vi "Teleop.vi"(10 "Match Info":T1={"Autonomous Elapsed Seconds"=0.0, "TeleOp Elapsed Seconds"=0.0, "Disabled Elapsed Seconds"=0.0, "Visited Autonomous"=FALSE, "Visited TeleOp"=FALSE, "Visited Disabled"=FALSE, "Autonomous Settings"={"Autonomous Style"=enum."Independent", "VI Refnum"=refnum}}, 11 "Call Context":T2) -> ()   [LabVIEW 2017]
doc: "This VI is called for each TeleOp packet received from the DS where the robot is not disabled. It is often used to read from the joysticks and update I/O or to update setpoints for timed control loops. It should complete and return within 20 milliseconds or it may miss DS packets."
uses:
  <vilib>/Rock Robotics/WPI/DriverStation/WPI_DriverStationDerivedRobotMode.ctl
  <vilib>/Rock Robotics/WPI/DriverStation/WPI_DriverStationMatch Info.ctl
  <vilib>/Rock Robotics/WPI/Utilities/WPI_GetSetVariantRefNum.vi
  <vilib>/Rock Robotics/Network Tables/NT Write Boolean Array.vi
  <vilib>/Rock Robotics/Network Tables/NT Write Numeric Array.vi
  <vilib>/Rock Robotics/Network Tables/NT Read Boolean.vi
  <vilib>/Rock Robotics/Network Tables/NT Read Number.vi
  Robot Global Data.vi
panel:
  out "Sample Slider 0":dbl(slide) scale=0.0..5.0
  out "Sample Boolean 1":bool
  out "Sample Boolean 0":bool
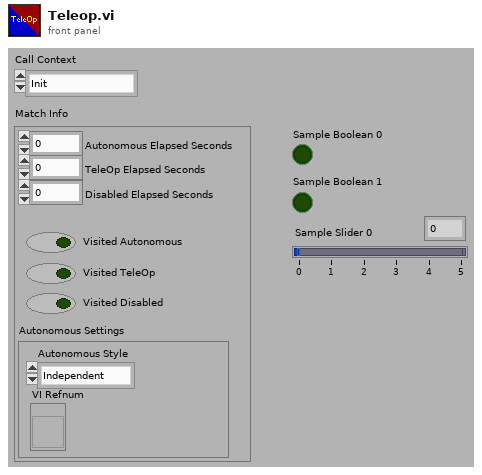
[diagram p1: front panel]
types:
  T1 = typedef "WPI_DriverStationMatch Info.ctl" = cluster{"Autonomous Elapsed Seconds":dbl, "TeleOp Elapsed Seconds":dbl, "Disabled Elapsed Seconds":dbl, "Visited Autonomous":bool, "Visited TeleOp":bool, "Visited Disabled":bool, "Autonomous Settings":cluster{"Autonomous Style":enum16{"Iterative", "Independent"}, "VI Refnum":refnum<vi>}}
  T2 = typedef "WPI_DriverStationDerivedRobotMode.ctl" = enum16{"Init", "Execute", "Stop"}
  T3 = enum16{"Linear", "Square  Root", "Square", "n^x"}
  T4 = typedef "WPI_JoystickDevRef.ctl" = cluster{"Device":T5}
  T5 = typedef "WPI_JoystickDeviceEnum.ctl" = enum16{"USB 0", "USB 1", "USB 2", "USB 3", "USB 4", "USB 5"}
  T6 = typedef "WPI_MotorControlDeviceRef.ctl" = cluster{"DeviceStatus":errorcluster, "Type":T7, "PWM":cluster{"PWM Channel":T8, "DeadBand":T9}, "CAN":cluster{"Device Number":u8, "SetOutput VI Ref":variant, "GetOutput VI Ref":variant, "Enable VI Ref":variant, "Disable VI Ref":variant, "Data":variant}, "Invert":bool, "DIO PWM":cluster{"PWM \"Enable\" Channel":T8, "DIOChannel":T10, "PWM Rate":dbl}}
  T7 = typedef "WPI_MotorControlType.ctl" = enum16{"PWM", "CAN", "DIO PWM"}
  T8 = typedef "FPGA_DIOPWMChannel.ctl" = enum8{"PWM 0", "PWM 1", "PWM 2", "PWM 3", "PWM 4", "PWM 5", "PWM 6", "PWM 7", "PWM 8", "PWM 9", "PWM MXP 0", "PWM MXP 1", "PWM MXP 2", "PWM MXP 3", "PWM MXP 4", "PWM MXP 5", "PWM MXP 6", "PWM MXP 7", "PWM MXP 8", "PWM MXP 9", "Invalid"}
  T9 = typedef "WPI_PWMDeadband.ctl" = cluster{"Name":string, "maxPositivePwm":i32, "minPositivePwm":i32, "centerPwm":i32, "maxNegativePwm":i32, "minNegativePwm":i32, "angularRange":u16}
  T10 = typedef "FPGA_DIOChannel.ctl" = enum8{"DIO 0", "DIO 1", "DIO 2", "DIO 3", "DIO 4", "DIO 5", "DIO 6", "DIO 7", "DIO 8", "DIO 9", "DIO MXP 0", "DIO MXP 1", "DIO MXP 2", "DIO MXP 3", "DIO MXP 4", "DIO MXP 5", "DIO MXP 6", "DIO MXP 7", "DIO MXP 8", "DIO MXP 9", "DIO MXP 10", "DIO MXP 11", "DIO MXP 12", "DIO MXP 13", "DIO MXP 14", "DIO MXP 15", "SPI Port CS1", "SPI Port CS2", "SPI Port CS3", "SPI Port MISO", "SPI Port MOSI", "Invalid"}
  T11 = cluster{"X":dbl, "Y":dbl, "Angle":dbl, "Magnitude":dbl}
  T12 = typedef "WPI_RobotDriveDevRef.ctl" = cluster{"DevStatus":errorcluster, "Motors[]":T6[], "Square Inputs":bool, "Max Output":dbl}
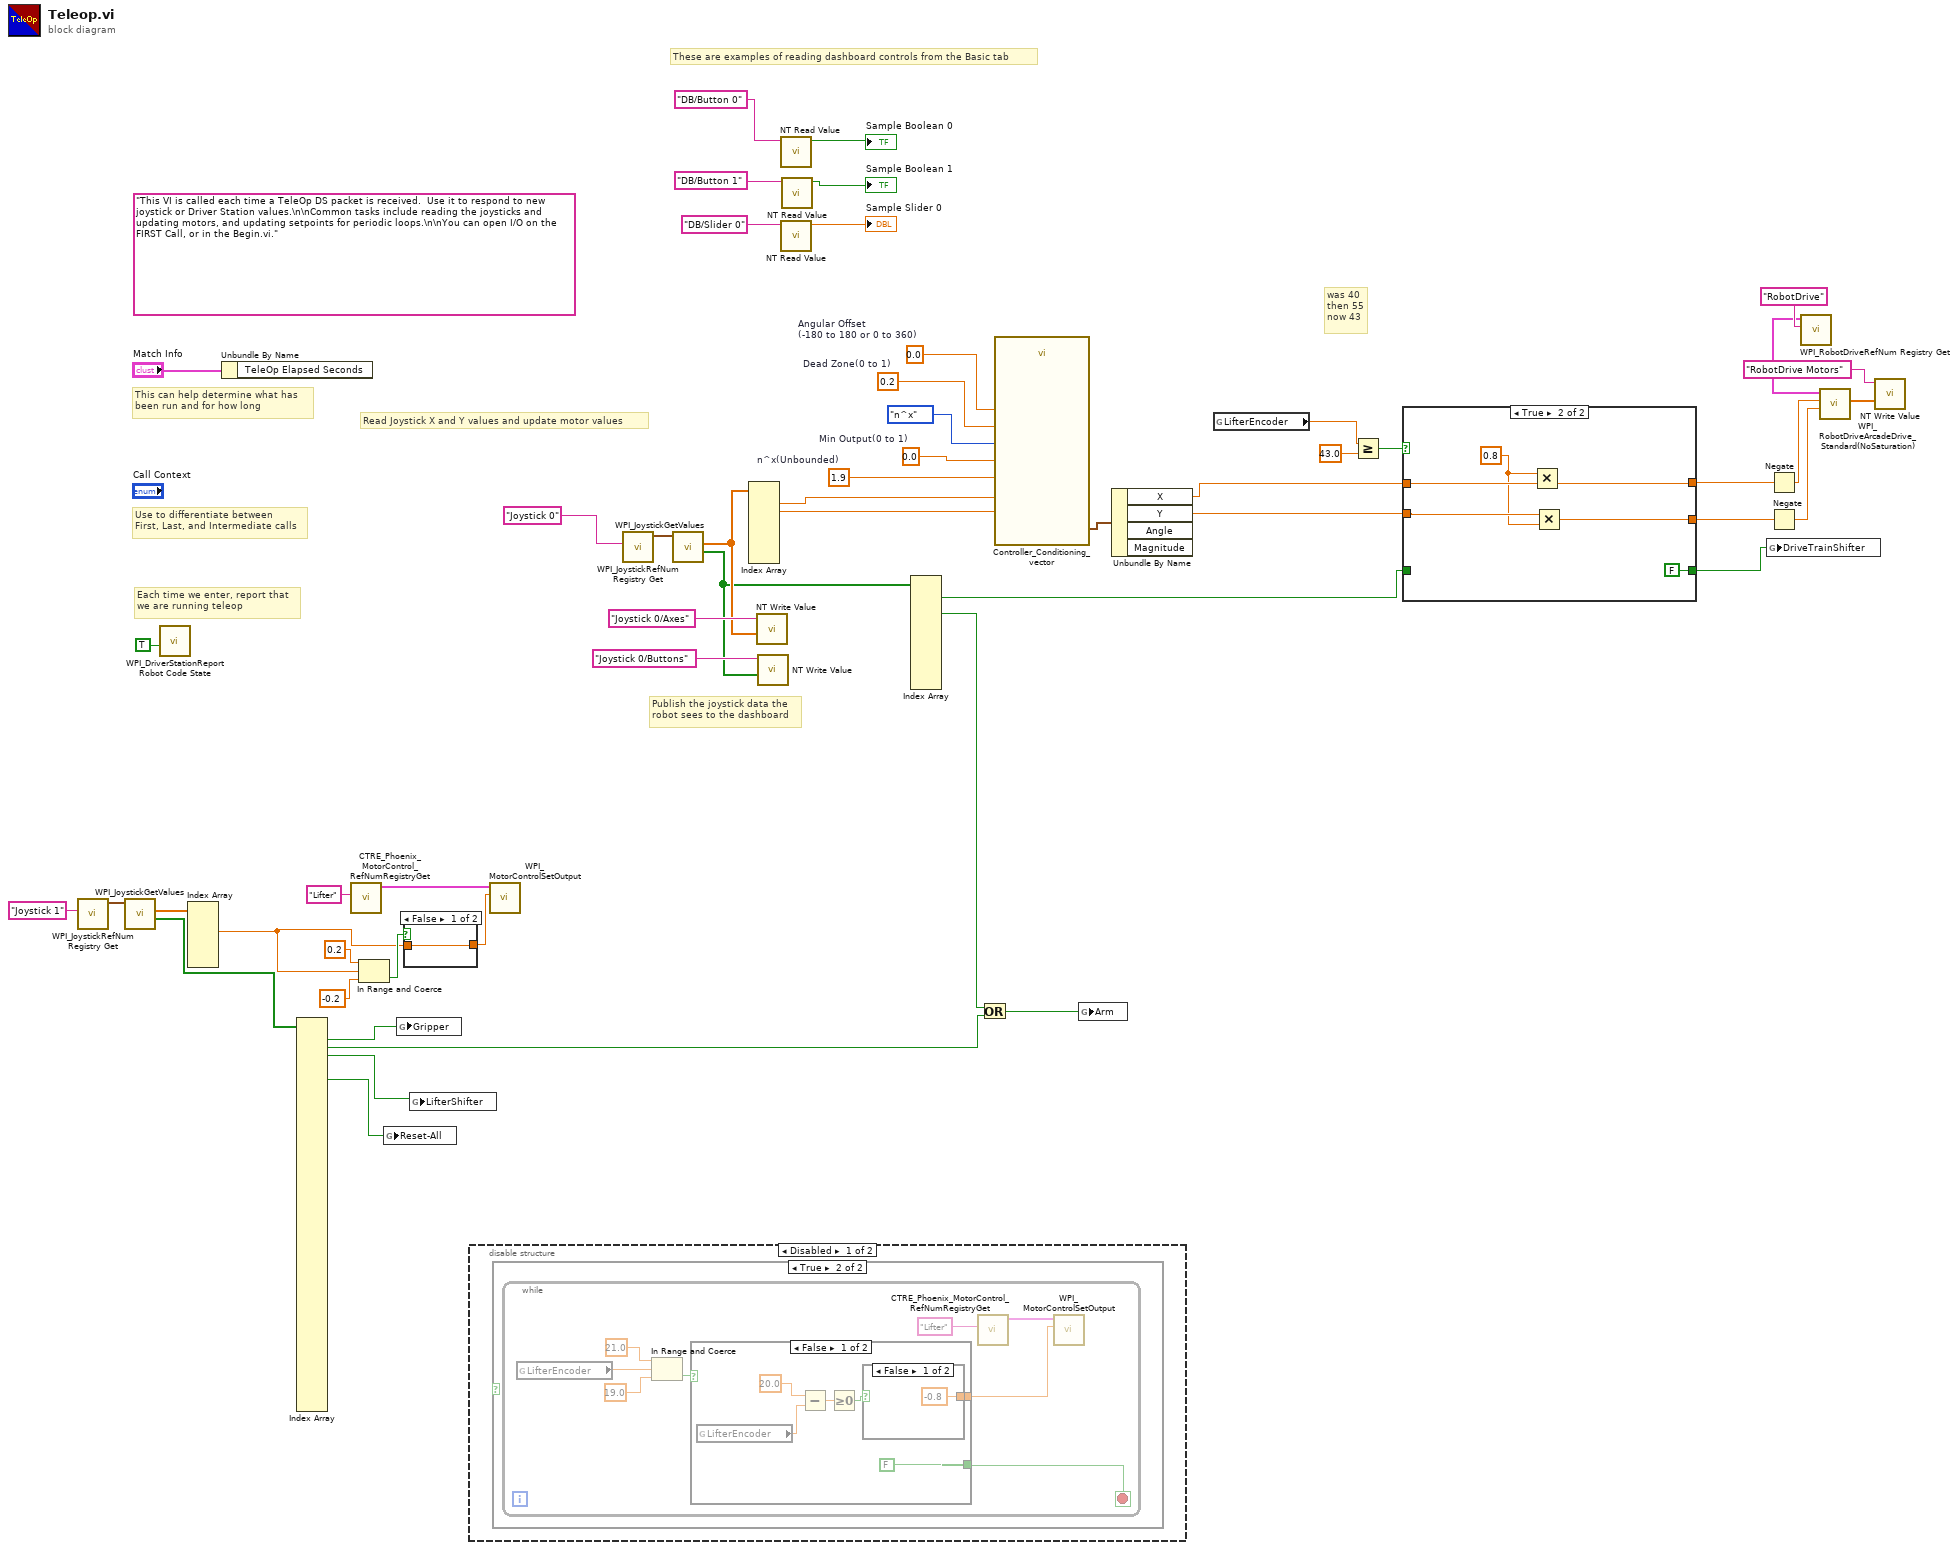
[diagram p0: block diagram]
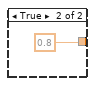
[diagram p4: hidden frame]
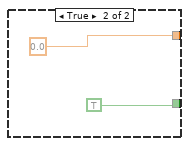
[diagram p5: hidden frame]
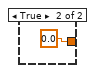
[diagram p7: hidden frame]
diagram:
  w13 = 1.9  # n^x(Unbounded)
  w14 = 0.0  # Min Output(0 to 1)
  w16 = 0.2  # Dead Zone(0 to 1)
  w17 = 0.0  # Angular Offset (-180 to 180 or 0 to 360)
  (unwired) "This VI is called each time a TeleOp DS packet is received.  Use it to respond to new joystick or Driver Station values.\n\nCommon tasks include reading the joysticks and updating motors, and updating setpoints for periodic loops.\n\nYou can open I/O on the FIRST Call, or in the Begin.vi."
  # "was 40\nthen 55\nnow 43"
  # "These are examples of reading dashboard controls from the Basic tab"
  # "Publish the joystick data the\nrobot sees to the dashboard"
  # "Each time we enter, report that\nwe are running teleop"
  # "Use to differentiate between\nFirst, Last, and Intermediate calls"
  # "This can help determine what has\nbeen run and for how long"
  # "Read Joystick X and Y values and update motor values"
  n1 = call <vilib>:"WPI_JoystickRefNum Registry Get.vi"("refnum name"="Joystick 1") -> ("JoystickDevRef"=w39:T4)  [unwired: 1 in, 9 out]
  n2 = call <vilib>:"WPI_JoystickGetValues.vi"("JoystickDevRef"=w39) -> ("Buttons"=w35:bool[], "Axes"=w38:dbl[])  [unwired: 6 in, 3 out]
  n3 = call <vilib>:"WPI_DriverStationReport Robot Code State.vi"("TeleOp"=TRUE ("Autonomous")) -> ()  [unwired: 10 in, 1 out]
  n4 = Index Array(array=w38) -> (element #2=w29:dbl)  [unwired: 6 in, 5 out]
  n5 = Unbundle By Name("Match Info") -> ()  [unwired: 1 out]
  n6 = Index Array(array=w35) -> (element #1=w28:bool, element #2=w26:bool, element #3=w10:bool, element #6=w11:bool)  [unwired: 47 in, 43 out]
  n7 = call <vilib>:"CTRE_Phoenix_MotorControl_RefNumRegistryGet.vi"("refnum name"="Lifter") -> ("PhoenixMotorControlDevRef"=w37:T6)  [unwired: 9 in, 1 out]
  n8 = In Range and Coerce(upper limit=0.2, x=w29, lower limit=-0.2) -> (In Range?=w31:bool)  [unwired: 1 out]
  n9 = global write "Robot Global Data.vi" "Reset-All"(w11) -> ()
  n10 = global write "Robot Global Data.vi" "Gripper"(w28) -> ()
  n11 = case shown="False" w31 {
    tunnel: [w55 0.0 ("Output")] -> w30
    tunnel: w29 -> [w55 _]
    frame False {
    }
    frame True {
    }
  }
  n12 = global write "Robot Global Data.vi" "LifterShifter"(w10) -> ()
  n13 = disable-structure shown="Disabled" {
    frame Disabled {
      n14 = case shown="True" {
        selector: _ -> [_ _]
        frame False {
          # "sohcahtoa"
        }
        frame True {
          n15 = while {
            stop <- w57 stop-if-true
            n16 = global read "Robot Global Data.vi" "LifterEncoder"() -> (w64:dbl)
            n17 = In Range and Coerce(upper limit=21.0, x=w64, lower limit=19.0) -> (In Range?=w61:bool)  [unwired: 1 out]
            n18 = case shown="False" w61 {
              tunnel: [w69 0.0] -> w58
              tunnel: [FALSE TRUE] -> w57
              frame False {
                n19 = global read "Robot Global Data.vi" "LifterEncoder"() -> (w68:dbl)
                n20 = Subtract(x=20.0, y=w68) -> (x-y=w66:dbl)
                n21 = Greater Or Equal To 0?(x=w66) -> (x >= 0?=w65:bool)
                n22 = case shown="False" w65 {
                  tunnel: [-0.8 0.8] -> w69
                  frame False {
                  }
                  frame True {
                  }
                }
              }
              frame True {
              }
            }
            n23 = call <vilib>:"CTRE_Phoenix_MotorControl_RefNumRegistryGet.vi"("refnum name"="Lifter") -> ("PhoenixMotorControlDevRef"=w60:T6)  [unwired: 9 in, 1 out]
            n24 = call <vilib>:"WPI_MotorControlSetOutput.vi"("Output"=w58, "MotorControlDevRef"=w60) -> ()  [unwired: 7 in, 3 out]
          }
        }
      }
    }
    frame Enabled {
    }
  }
  n25 = call <vilib>:"WPI_MotorControlSetOutput.vi"("Output"=w30, "MotorControlDevRef"=w37) -> ()  [unwired: 7 in, 3 out]
  n26 = call <vilib>:"WPI_JoystickRefNum Registry Get.vi"("refnum name"="Joystick 0") -> ("JoystickDevRef"=w52:T4)  [unwired: 1 in, 9 out]
  n27 = call <vilib>:"WPI_JoystickGetValues.vi"("JoystickDevRef"=w52) -> ("Buttons"=w41:bool[], "Axes"=w48:dbl[])  [unwired: 6 in, 3 out]
  n28 = Index Array(array=w48) -> (element #1=w19:dbl, element #2=w18:dbl)  [unwired: 8 in, 6 out]
  n29 = call-poly <vilib>:"NT Write Value.vi"("Numeric Array"=w48, "Name"="Joystick 0/Axes") -> ()  [unwired: 9 in, 1 out]
  n30 = call-poly <vilib>:"NT Write Value.vi"("Boolean Array"=w41, "Name"="Joystick 0/Buttons") -> ()  [unwired: 9 in, 1 out]
  n31 = call-poly <vilib>:"NT Read Value.vi"("Name"="DB/Button 0" ("refnum name")) -> ("Boolean"=→"Sample Boolean 0":bool)  [unwired: 9 in, 1 out]
  n32 = call-poly <vilib>:"NT Read Value.vi"("Name"="DB/Slider 0" ("refnum name")) -> ("Numeric"=→"Sample Slider 0":dbl)  [unwired: 9 in, 1 out]
  n33 = call-poly <vilib>:"NT Read Value.vi"("Name"="DB/Button 1" ("refnum name")) -> ("Boolean"=→"Sample Boolean 1":bool)  [unwired: 9 in, 1 out]
  n34 = Index Array(array=w41) -> (element #1=w1:bool, element #3=w34:bool)  [unwired: 12 in, 10 out]
  n35 = Or(x=w34, y=w26) -> (x .or. y?=w27:bool)
  n36 = call "Controller_Conditioning_vector.vi"("Angular Offset\n(-180 to 180 or 0 to 360)"=w17, "Min Output(0 to 1)"=w14, "n^x(Unbounded)"=w13, "Enum"=T3."n^x", "Dead Zone(0 to 1)"=w16, "Y(-1 to 1)"=w18, "X(-1 to 1)"=w19) -> ("output cluster"=w12:T11)  [unwired: 4 in]
  n37 = global write "Robot Global Data.vi" "Arm"(w27) -> ()
  n38 = Unbundle By Name(w12) -> ("X"=w6:dbl, "Y"=w8:dbl)  [unwired: 2 out]
  n39 = global read "Robot Global Data.vi" "LifterEncoder"() -> (w5:dbl)
  n40 = Greater Or Equal?(x=w5, y=43.0) -> (x >= y?=w4:bool)
  n41 = case shown="True" w4 {
    tunnel: [w77 w82] -> w9
    tunnel: w8 -> [w77 w83]
    tunnel: [w76 w80] -> w7
    tunnel: w6 -> [w76 w81]
    tunnel: [w75 FALSE] -> w2
    tunnel: w1 -> [w75 _]
    frame False {
    }
    frame True {
      w79 = 0.8 ("upper limit")
      n42 = Multiply(x=w79, y=w81) -> (x*y=w80:dbl)
      n43 = Multiply(x=w83, y=w79) -> (x*y=w82:dbl)
    }
  }
  n44 = global write "Robot Global Data.vi" "DriveTrainShifter"(w2) -> ()
  n45 = Negate(x=w7) -> (-x=w21:dbl)
  n46 = Negate(x=w9) -> (-x=w20:dbl)
  n47 = call <vilib>:"WPI_RobotDriveRefNum Registry Get.vi"("refnum name"="RobotDrive") -> ("RobotDriveDevRef"=w24:T12)  [unwired: 1 in, 9 out]
  n48 = call <vilib>:"WPI_RobotDriveArcadeDrive_Standard(NoSaturation).vi"("Y axis value"=w20, "X axis value"=w21, "RobotDriveDevRef"=w24) -> ("Motor Values"=w23:dbl[])  [unwired: 1 in, 7 out]
  n49 = call-poly <vilib>:"NT Write Value.vi"("Numeric Array"=w23, "Name"="RobotDrive Motors") -> ()  [unwired: 9 in, 1 out]
